vi "write wait.vi"(8 "error in (no error)":errorcluster caption="entrée d'erreur (pas d'erreur)", 11 "DelayLineLS4 en entrée":refnum<class "DLLS4.lvclass">) -> (0 "error out":errorcluster caption="sortie d'erreur", 3 "DelayLineLS4 en sortie":refnum<class "DLLS4.lvclass">)   [LabVIEW 2020]
uses:
  DLLS4.lvclass
  C:/dev/TRANCON/Classes/Delay Line/DelayLine.lvclass
  C:/dev/TRANCON/Classes/GeneralFunctionality/GeneralFunctionality.lvclass
  GeneralFunctionality/GeneralFunctionality.lvclass/GeneralFunctionality.ctl
  DelayLine.lvclass/DelayLine.ctl
  Config/Config.lvclass
  GeneralFunctionality/GeneralFunctionality.lvclass
  DelayLine.lvclass
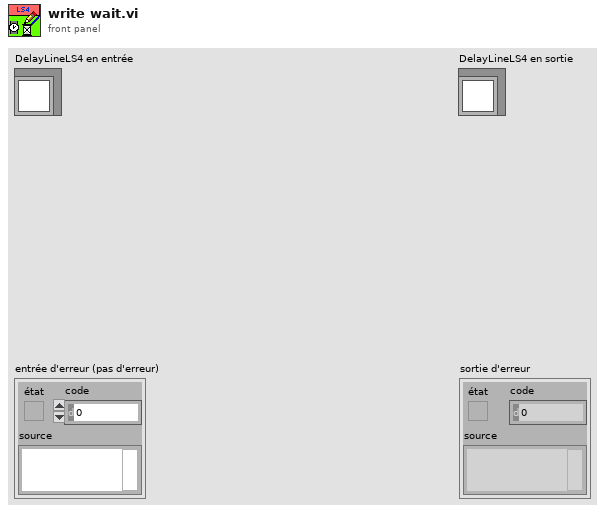
[diagram p1: front panel]
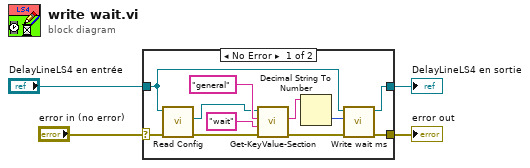
[diagram p0: block diagram]
diagram:
  n1 = case shown="No Error" "error in (no error)" {
    selector: "error in (no error)" -> [w15 w16]
    tunnel: [w8 w16] -> w3
    tunnel: [w7 w17] -> w1
    tunnel: "DelayLineLS4 en entrée" -> [w6 w17]
    frame No Error {
      n2 = call "Read Config.vi"("error in (no error)"=w15, "GeneralFunctionality en entrée"=w6) -> ("error out"=w14:errorcluster, "Config.lvclass"=w11:refnum<class "Config.lvclass">)  [unwired: 7 in, 1 out]
      n3 = call-dynamic "Get-KeyValue-Section.vi"("error in (no error)"=w14, "Key"="wait", "Section"="general", "Config in"=w11) -> ("error out"=w9:errorcluster, "Value"=w10:string)  [unwired: 5 in, 1 out]
      n4 = Decimal String To Number(string=w10) -> (number=w5:i32)  [unwired: 2 in, 1 out]
      n5 = call "Write wait ms.vi"("error in (no error)"=w9, "wait ms"=w5, "DelayLine in"=w6) -> ("error out"=w8:errorcluster, "DelayLine out"=w7:refnum<class "DLLS4.lvclass">)  [unwired: 7 in]
    }
    frame Error {
    }
  }
  "error out" <- w3
  "DelayLineLS4 en sortie" <- w1
